vi "SVL Set dB Reference.vi"   [LabVIEW 2017]
doc: "Sets the specified <B>dB reference [EU]</B> as an attribute in the <B>scaled signal out [EU]</B> waveform. <B>dB reference [EU]</B> is used for all downstream conversions to dB. Wire data to the <B>scaled signal in [EU]</B> input to determine the polymorphic instance to use or manually select the instance."
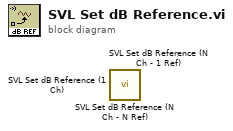
[diagram p0: block diagram]
diagram:
  n1 = call <vilib>:"SVL Set dB Reference (N Ch - N Ref).vi"() -> ()  [unwired: 10 in, 2 out]
  n2 = call <vilib>:"SVL Set dB Reference (N Ch - 1 Ref).vi"() -> ()  [unwired: 10 in, 2 out]
  n3 = call <vilib>:"SVL Set dB Reference (1 Ch).vi"() -> ()  [unwired: 10 in, 2 out]
